vi "Pie Chart.vi"(9 "Draw Area Size":T1, 11 "Array":cluster{"Label":string, "Value":dbl}[](array[cluster])=[{"Label"="This", "Value"=23.0}, {"Label"="is", "Value"=13.0}, {"Label"="only", "Value"=36.0}, {"Label"="a", "Value"=7.0}, {"Label"="test", "Value"=21.0}]) -> (3 "Picture":picture)   [LabVIEW 2016, in "CML UI.lvlib" / "Circular Cue Helper.lvlib"]
doc: "This VI generates a pie chart using the LabVIEW picture control. Given an array of clusters containing a label and a value, a pie chart with legend is generated and displayed."
uses:
  Circular Cue Helper.lvlib
  <vilib>/Utility/miscctls.llb/LVBoundsTypeDef.ctl
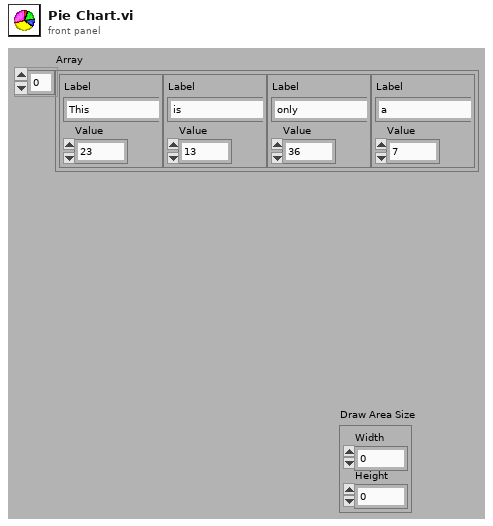
[diagram p1: front panel]
types:
  T1 = typedef "LVBoundsTypeDef.ctl" = cluster{"Width":u32, "Height":u32}
  T2 = cluster{"left":i16, "top":i16, "right":i16, "bottom":i16}
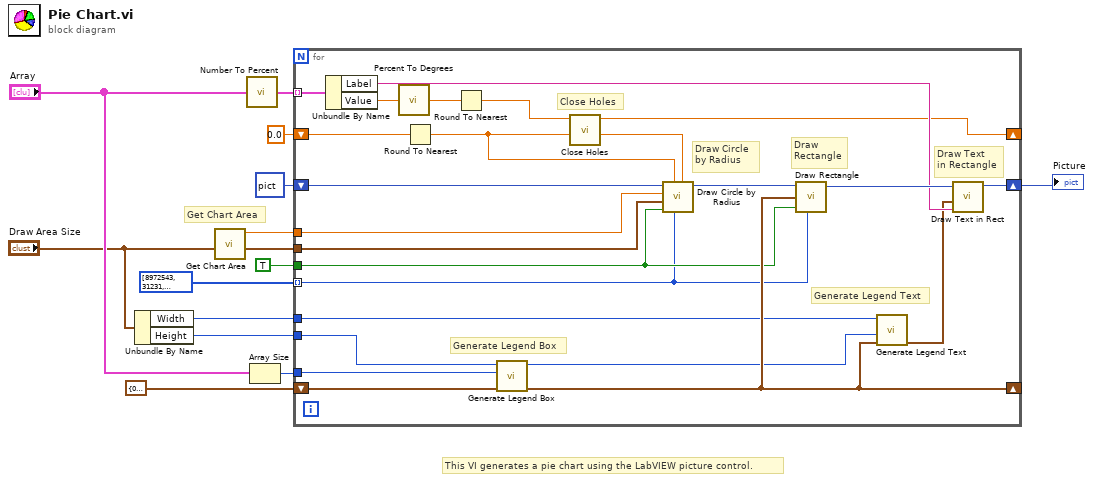
[diagram p0: block diagram]
diagram:
  # "This VI generates a pie chart using the LabVIEW picture control."
  # "Get Chart Area"
  n1 = Unbundle By Name("Draw Area Size") -> ("Width"=w9:u32, "Height"=w11:u32)
  n2 = call "Get Chart Area.vi"("Draw Area Size"="Draw Area Size") -> ("Chart Area Size"=w1:cluster{"Width":dbl, "Height":dbl}, "Height"=w3:dbl)  [unwired: 9 in]
  n3 = call "Number To Percent.vi"("Array In"="Array") -> ("Array Out"=w6:cluster{"Label":string, "Value":dbl}[])
  n4 = Array Size(array="Array") -> (size(s)=w5:i32)
  n5 = for {
    tunnel: w6 -> [w37] mode=indexing
    shift-right: [w28] -> w12
    shift-left: picture data[5B] ("new picture") -> [w36]
    tunnel: w3 -> [w32]
    shift-right: [w17] -> _
    shift-left: 0.0 -> [w21]
    tunnel: u32[] [8972543, 31231, 327900, 441827, 16512, 2768895, 11121611, 7171459, 0] -> [w24] mode=indexing
    shift-right: [w38] -> _
    shift-left: T2 {"left"=0, "top"=0, "right"=0, "bottom"=0} ("rect") -> [w33]
    tunnel: w11 -> [w31]
    tunnel: TRUE ("fill?(F)") -> [w30]
    tunnel: w9 -> [w25]
    tunnel: w5 -> [w22]
    tunnel: w1 -> [w15]
    # "Draw Circle \nby Radius"
    # "Draw Text\nin Rectangle"
    # "Draw \nRectangle"
    # "Close Holes"
    # "Generate Legend Text"
    # "Generate Legend Box"
    n6 = Unbundle By Name(w37) -> ("Label"=w27:string, "Value"=w35:dbl)
    n7 = call "Percent To Degrees.vi"("Percent"=w35) -> ("Degrees"=w19:dbl)
    n8 = Round To Nearest(number=w21) -> (nearest integer value=w20:dbl)
    n9 = Round To Nearest(number=w19) -> (nearest integer value=w16:dbl)
    n10 = call "Generate Legend Box.vi"("rect 2"=w33, "Array Size"=w22, "Height"=w31) -> ("rect"=w38:T2, "Gap"=w23:i32)  [unwired: 7 in]
    n11 = call "Close Holes.vi"("Start Angle"=w20, "Preliminary Arc Size"=w16) -> ("Final Arc Size"=w18:dbl, "Final Angle"=w17:dbl)  [unwired: 8 out]
    n12 = call <vilib>:"Draw Circle by Radius.vi"("arc size(360)"=w18, "color(black)"=w24, "start angle(0)"=w20, "fill?(F)"=w30, "pixel center"=w15, "radius"=w32, "picture"=w36) -> ("new picture"=w34:picture)  [unwired: 1 in, 3 out]
    n13 = call <vilib>:"Draw Rectangle.vi"("picture"=w34, "rect"=w38, "fill?(F)"=w30, "color(black)"=w24) -> ("new picture"=w29:picture)  [unwired: 5 in]
    n14 = call "Generate Legend Text.vi"("Last Text"=w38, "Gap"=w23, "Width"=w25) -> ("New Text"=w26:T2)  [unwired: 8 in]
    n15 = call <vilib>:"Draw Text in Rect.vi"("text"=w27, "rect"=w26, "picture"=w29) -> ("new picture"=w28:picture)  [unwired: 5 in, 3 out]
  }
  "Picture" <- w12
